vi "Image_Processing_Queue.vi"(5 "Data":T4={"system"={"info"={"menuSelect"=0, "version"=0, "serial"="Test Sample", "captureActive"=FALSE, "captureBegin"=FALSE, "emptyAndRefill"=FALSE}, "userInfo"={"operatorName"="", "date"=timestamp(2713993200 s since 1904-01-01)}, "camera"={"exposureTime"=0, "aperture"=enum."Item 0", "framerate"=0, "framerateMax"=500, "legacyAttributes"=FALSE}}, "connections"={"arduino"={"connection"="MRJ", "status"=FALSE, "openState"=FALSE, "emptyStart"=0}, "pump"={"connection"="MRJ", "status"=FALSE, "command"="", "dispenseSpeed"=100, "flushSize"=100}, "camera"={"cam1"={"connection"="", "status"=FALSE}, "cam2"={"connection"="", "status"=FALSE}}}, "queue"={"process"={"cam1"=refnum, "cam2"=refnum, "queueSize"=0}, "save"={"cam1"=refnum, "cam2"=refnum, "queueSize"=0}, "overloadThreshold"=0}, "imageProcess"={"cam1"={"preAllocation"={"image"="Station", "originalDisplay"="Station", "originalRgb"="Station", "binary"="Station", "save"="Station", "calibrationFull"=refnum, "calibrationDetect"=refnum}, "calibration"={"pathFull"=path "C:/Users/au540322/Desktop/IHS_Project/images/Debris/Debris_0/Debris_0_2019_06_01-23-32-49-686.PNG", "pathDetect"=path "C:/Users/au540322/Desktop/IHS_Project/images/Debris/Debris_0/Debris_0_2019_06_01-23-32-49-686.PNG", "ROI"={"Left"=0, "Top"=0, "Right"=0, "Bottom"=0, "Rotation"=0.0}}}, "cam2"={"preAllocation"={"image"=refnum, "originalDisplay"=refnum, "originalRgb"=refnum, "binary"=refnum, "save"=refnum, "calibrationFull"=refnum, "calibrationDetect"=refnum}, "calibration"={"pathFull"=path "C:/Users/au540322/Desktop/IHS_Project/images/Debris/Debris_0/Debris_0_2019_06_01-23-32-49-686.PNG", "pathDetect"=path "C:/Users/au540322/Desktop/IHS_Project/images/Debris/Debris_0/Debris_0_2019_06_01-23-32-49-686.PNG", "ROI"={"Left"=0, "Top"=0, "Right"=0, "Bottom"=0, "Rotation"=0.0}}}, "process"={"planeExtract"=refnum, "planeSubtract"=refnum, "cropMask"=refnum}, "detection"={"sampleTimeout"=500, "sizeThreshold"=500, "detectionRegionPct"=0.0}}, "sampleData"={"sampleId"="", "projectId"="", "voucherID"="", "speciesName"="", "collectionDate"=timestamp(2713993200 s since 1904-01-01), "sampleStation"="", "location"="", "lat"=0.0, "lon"=0.0, "determiner"="", "sex"="", "otherNotes"=""}, "Session In"=""} {"sampleData"."collectionDate" format="%<%Y-%m-%d>T"; "imageProcess"."detection"."sizeThreshold" min=1; "imageProcess"."cam2"."calibration"."ROI"."Rotation" format="%.2f"; "imageProcess"."cam2"."calibration"."ROI"."Left" scale=0.0..1024.0; "imageProcess"."cam2"."calibration"."ROI"."Right" scale=0.0..1024.0; "imageProcess"."cam1"."calibration"."ROI"."Rotation" format="%.2f"; "imageProcess"."cam1"."calibration"."ROI"."Left" scale=0.0..1024.0; "imageProcess"."cam1"."calibration"."ROI"."Right" scale=0.0..1024.0; "queue"."overloadThreshold" min=1; "queue"."save"."queueSize" min=1; "queue"."process"."queueSize" min=1; "connections"."pump"."flushSize" min=1; "connections"."pump"."dispenseSpeed" min=1; "system"."camera"."framerateMax" min=1; "system"."userInfo"."date" format="%<%Y-%m-%dT%H:%M:%S+%z>T"; "system"."info"."version" items=["Standard", "XL"]; "system"."info"."menuSelect" items=["Session Data", "Extended Setup", "Buffer", "Camera", "Dispenser", "Stats", "Connections"]}) -> (10 "Status":T1, 11 "Detection error":errorcluster, 12 "Process queue":T2, 13 "Last Image?":bool, 14 "Object1":T3, 15 "Object2":T3, 16 "Image 1":T3, 17 "Image 2":T3, 18 "Binary 1":T3, 19 "Binary 2":T3)   [LabVIEW 2022 SP3]
doc: "Saves every 6th image in a sub folder in the current directory (specified from Sample Name). When a true is sent to Sample+1 a new subfolder is created with incremental numbering.\nExample of folders: \n../images/Sample_Name/Sample_Name1\n../images/Sample_Name/Sample_Name2"
uses:
  controls/Data.ctl
  <vilib>/userdefined/High Color/IMAQdx.ctl
  <vilib>/vision/Image Controls.llb/IMAQ Image.ctl
  <extravilib>/ChannelInstances/Tag-c(bool,bool)/))Channel.ctl
  Camera_ID.ctl
  <extravilib>/ChannelInstances/Tag-c(bool,bool)/Write With Abort.vi
  <extravilib>/ChannelInstances/Tag-c(bool,bool)/Endpoint.vi
  <extravilib>/ChannelInstances/Tag-c(bool,bool).lvlib
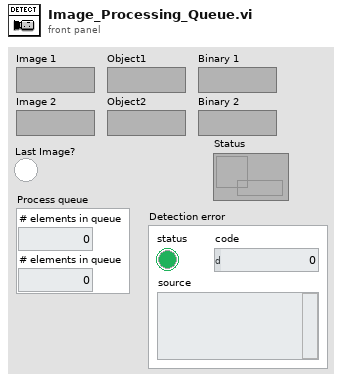
[diagram p1: front panel]
types:
  T1 = typedef "Tag-c(bool,bool).lvlib/))Channel.ctl" = refnum<queue>
  T2 = cluster{"# elements in queue":i32, "# elements in queue":i32}
  T3 = typedef "IMAQ Image.ctl" = refnum<image>
  T4 = typedef "Data.ctl" = cluster{"system":cluster{"info":cluster{"menuSelect":u16, "version":u16, "serial":string, "captureActive":bool, "captureBegin":bool, "emptyAndRefill":bool}, "userInfo":cluster{"operatorName":string, "date":timestamp}, "camera":cluster{"exposureTime":i32, "aperture":enum32{"Item 0", "Item 1", "Item 2", "Item 3"}, "framerate":i32, "framerateMax":i32, "legacyAttributes":bool}}, "connections":cluster{"arduino":cluster{"connection":refnum<visa-resource-name>, "status":bool, "openState":bool, "emptyStart":u32}, "pump":cluster{"connection":refnum<visa-resource-name>, "status":bool, "command":string, "dispenseSpeed":i32, "flushSize":i32}, "camera":cluster{"cam1":cluster{"connection":T5, "status":bool}, "cam2":cluster{"connection":T5, "status":bool}}}, "queue":cluster{"process":cluster{"cam1":refnum<queue>, "cam2":refnum<queue>, "queueSize":i32}, "save":cluster{"cam1":refnum<queue>, "cam2":refnum<queue>, "queueSize":i32}, "overloadThreshold":i32}, "imageProcess":cluster{"cam1":cluster{"preAllocation":cluster{"image":T3, "originalDisplay":T3, "originalRgb":T3, "binary":T3, "save":T3, "calibrationFull":T3, "calibrationDetect":T3}, "calibration":cluster{"pathFull":path, "pathDetect":path, "ROI":T6}}, "cam2":cluster{"preAllocation":cluster{"image":T3, "originalDisplay":T3, "originalRgb":T3, "binary":T3, "save":T3, "calibrationFull":T3, "calibrationDetect":T3}, "calibration":cluster{"pathFull":path, "pathDetect":path, "ROI":T6}}, "process":cluster{"planeExtract":T3, "planeSubtract":T3, "cropMask":T3}, "detection":cluster{"sampleTimeout":i32, "sizeThreshold":i32, "detectionRegionPct":dbl}}, "sampleData":cluster{"sampleId":string, "projectId":string, "voucherID":string, "speciesName":string, "collectionDate":timestamp, "sampleStation":string, "location":string, "lat":dbl, "lon":dbl, "determiner":string, "sex":string, "otherNotes":string}, "Session In":T5}
  T5 = typedef "IMAQdx.ctl" = refnum<k21>
  T6 = typedef "IMAQ Rectangle" = cluster{"Left":i32, "Top":i32, "Right":i32, "Bottom":i32, "Rotation":dbl}
  T7 = typedef "Camera_ID.ctl" = enum16{"Camera 1", "Camera 2"}
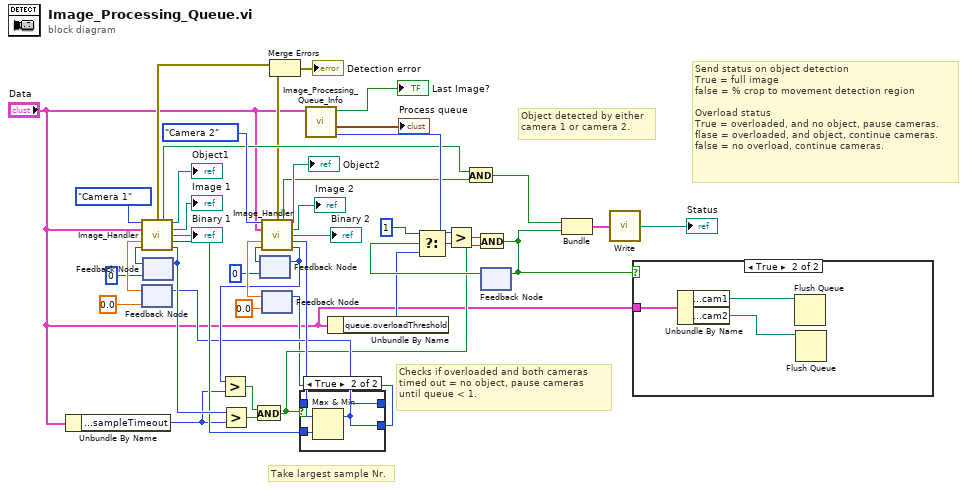
[diagram p0: block diagram]
diagram:
  # "Take largest sample Nr."
  # "Send status on object detection\nTrue = full image\nfalse = % crop to movement detection region\n\nOverload status\nTrue = overloaded, and no object, pause cameras.\nflase = overloaded, and object, continue cameras.\nfalse = no overload, continue cameras."
  # "Object detected by either\ncamera 1 or camera 2."
  # "Checks if overloaded and both cameras \ntimed out = no object, pause cameras \nuntil queue < 1."
  n1 = Unbundle By Name("Data") -> ("imageProcess.detection.sampleTimeout"=w22:i32)
  n2 = feedback #1(0.0 ("Sample nr")) -> (w35:dbl)
  n3 = feedback #2(0 ("Timeout out")) -> (w33:i32)
  n4 = call "Image_Handler.vi"("Camera"=Camera_ID."Camera 1", "Data"="Data", "Prev. sample"=w35, "Timeout in"=w33) -> ("Detection error"=w7:errorcluster, "Object"=w11:bool, "Detected object"=→"Object1":T3, "Image Out"=→"Image 1":T3, "Binary"=→"Binary 1":T3, "Sample nr"=w25:i32, "Timeout out"=w27:i32)  [unwired: 5 in]
  n5 = feedback-in #2(w27) -> ()
  n6 = Greater?(x=w27, y=w22) -> (0:w24:bool)
  n7 = feedback #3(0 ("Timeout out")) -> (w32:i32)
  n8 = feedback #4(0.0 ("Sample nr")) -> (w34:dbl)
  n9 = call "Image_Handler.vi"("Camera"=Camera_ID."Camera 2", "Data"="Data", "Prev. sample"=w34, "Timeout in"=w32) -> ("Detection error"=w8:errorcluster, "Object"=w12:bool, "Detected object"=→"Object2":T3, "Image Out"=→"Image 2":T3, "Binary"=→"Binary 2":T3, "Sample nr"=w26:i32, "Timeout out"=w23:i32)  [unwired: 5 in]
  n10 = Greater?(x=w23, y=w22) -> (0:w21:bool)
  n11 = And(x=w21, y=w24) -> (x .and. y?=w4:bool)
  n12 = feedback-in #3(w23) -> ()
  n13 = Merge Errors(w7, w8) -> (→"Detection error":errorcluster)
  n14 = case shown="True" w4 {
    tunnel: w26 -> [w45 w49]
    tunnel: w25 -> [w46 w48]
    tunnel: [w46 w47] -> w5
    tunnel: [w45 w47] -> w3
    frame False {
    }
    frame True {
      n15 = Max & Min(x=w49, y=w48) -> (max(x,y)=w47:i32)  [unwired: 1 out]
    }
  }
  n16 = feedback-in #1(w5) -> ()
  n17 = feedback-in #4(w3) -> ()
  n18 = call "Image_Processing_Queue_Info.vi"("Data"="Data") -> ("Max Queue Size"=w15:i32, "Queue data"=→"Process queue":T2, "Last Image?"=→"Last Image?":bool)  [unwired: 8 in]
  n19 = Unbundle By Name("Data") -> ("queue.overloadThreshold"=w14:i32)
  n20 = And(x=w11, y=w12) -> (x .and. y?=w13:bool)
  n21 = feedback #5() -> (w17:bool)  [unwired: 1 in]
  n22 = Select(t=1 ("y"), s=w17, f=w14) -> (s? t:f=w16:i32)
  n23 = Greater?(x=w15, y=w16) -> (0:w19:bool)
  n24 = And(x=w19, y=w4) -> (x .and. y?=w2:bool)
  n25 = feedback-in #5(w2) -> ()
  n26 = Bundle(w13, w2) -> (w10:cluster{bool, bool})  [unwired: 1 in]
  n27 = call <extravilib>:"Write.vi"("element"=w10) -> ("channel"=→"Status":T1)  [unwired: 1 out]
  n28 = case shown="True" w2 {
    tunnel: "Data" -> [_ w52]
    frame False {
    }
    frame True {
      n29 = Unbundle By Name(w52) -> ("queue.process.cam1"=w51:refnum<queue>, "queue.process.cam2"=w50:refnum<queue>)
      n30 = Flush Queue(queue=w51) -> ()  [unwired: 1 in, 3 out]
      n31 = Flush Queue(queue=w50) -> ()  [unwired: 1 in, 3 out]
    }
  }
